vi "knownhosts_add.vi"() -> ()   [LabVIEW 2013]
doc: "Illustrates how to add a known host to the collection of known hosts."
uses:
  libssh2/libssh2_knownhost.ctl
  libssh2/Known Host Refnum.ctl
  libssh2/libssh2_init_default.vi
  libssh2/libssh2.lvlib
panel:
  out "error out":errorcluster
  out "known hosts":T1[](array[typedef])
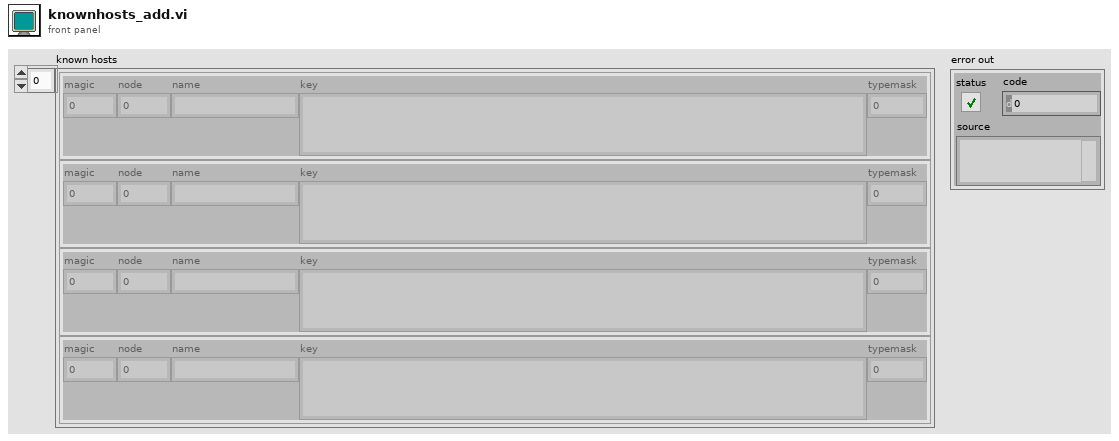
[diagram p1: front panel]
types:
  T1 = typedef "libssh2.lvlib/libssh2_knownhost.ctl" = cluster{"magic":u32, "node":u64, "name":string, "key":string, "typemask":i32}
  T2 = typedef "libssh2.lvlib/Known Host Refnum.ctl" = refnum<k1>
  T3 = typedef "libssh2.lvlib/Session Refnum.ctl" = refnum<k1>
  T4 = typedef "libssh2.lvlib/Known Host Collection Refnum.ctl" = refnum<k1>
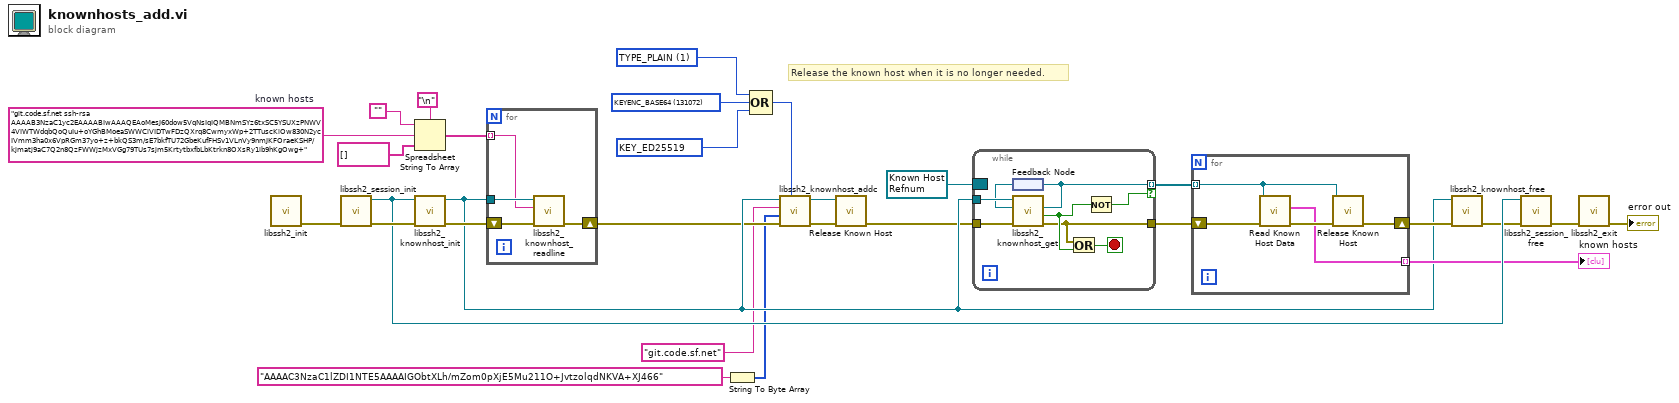
[diagram p0: block diagram]
diagram:
  w2 = 1835008 items=["TYPE_PLAIN"=1, "TYPE_SHA1"=2, "TYPE_CUSTOM"=3, "KEYENC_RAW"=65536, "KEYENC_BASE64"=131072, "KEY_RSA1"=262144, "KEY_SSHRSA"=524288, "KEY_SSHDSS"=786432, "KEY_ECDSA_256"=1048576, "KEY_ECDSA_384"=1310720, "KEY_ECDSA_521"=1572864, "KEY_ED25519"=1835008, "KEY_UNKNOWN"=3932160] ("typemask")
  w3 = 131072 items=["TYPE_PLAIN"=1, "TYPE_SHA1"=2, "TYPE_CUSTOM"=3, "KEYENC_RAW"=65536, "KEYENC_BASE64"=131072, "KEY_RSA1"=262144, "KEY_SSHRSA"=524288, "KEY_SSHDSS"=786432, "KEY_ECDSA_256"=1048576, "KEY_ECDSA_384"=1310720, "KEY_ECDSA_521"=1572864, "KEY_ED25519"=1835008, "KEY_UNKNOWN"=3932160] ("typemask")
  w4 = 1 items=["TYPE_PLAIN"=1, "TYPE_SHA1"=2, "TYPE_CUSTOM"=3, "KEYENC_RAW"=65536, "KEYENC_BASE64"=131072, "KEY_RSA1"=262144, "KEY_SSHRSA"=524288, "KEY_SSHDSS"=786432, "KEY_ECDSA_256"=1048576, "KEY_ECDSA_384"=1310720, "KEY_ECDSA_521"=1572864, "KEY_ED25519"=1835008, "KEY_UNKNOWN"=3932160] ("typemask")
  w19 = "git.code.sf.net ssh-rsa AAAAB3NzaC1yc2EAAAABIwAAAQEAoMesJ60dow5VqNsIqIQMBNmSYz6txSC5YSUXzPNWV4VIWTWdqbQoQuIu+oYGhBMoeaSWWCiVIDTwFDzQXrq8CwmyxWp+2TTuscKiOw830N2ycIVmm3ha0x6VpRGm37yo+z+bkQS3m/sE7bkfTU72GbeKufFHSv1VLnVy9nmJKFOraeKSHP/kjmatj9aC7Q2n8QzFWWjzMxVGg79TUs7sjm5KrtytbxfbLbKtrkn8OXsRy1ib9hKgOwg+"  # known hosts
  w21 = T2 refnum items=["Host"] ("next")
  # "Release the known host when it is no longer needed."
  n1 = call-poly "libssh2_init.vi"() -> ("error out"=w29:errorcluster)  [unwired: 11 in]
  n2 = call "libssh2_session_init.vi"("error in (no error)"=w29) -> ("error out"=w28:errorcluster, "session"=w27:T3)  [unwired: 9 in]
  n3 = Spreadsheet String To Array(delimiter (Tab)="\n", format string="", spreadsheet string=w19, array type (2D Dbl)=string[] []) -> (array=w18:string[])
  n4 = call "libssh2_knownhost_init.vi"("error in (no error)"=w28, "session"=w27) -> ("error out"=w24:errorcluster, "known hosts collection"=w11:T4)  [unwired: 8 in]
  n5 = for {
    tunnel: w11 -> [w31]
    tunnel: w18 -> [w30] mode=indexing
    shift-right: [w32] -> w10
    shift-left: w24 -> [w33]
    n6 = call "libssh2_knownhost_readline.vi"("error in (no error)"=w33, "line"=w30, "known hosts collection"=w31) -> ("error out"=w32:errorcluster)  [unwired: 8 in]
  }
  n7 = String To Byte Array(string="AAAAC3NzaC1lZDI1NTE5AAAAIGObtXLh/mZom0pXjE5Mu211O+JvtzolqdNKVA+XJ466" ("hostname")) -> (unsigned byte array=w7:u8[])
  n8 = Compound Arithmetic op=OR(w4, w3, w2) -> (w1:i32)
  n9 = call "libssh2_knownhost_addc.vi"("typemask"=w1, "error in (no error)"=w10, "key"=w7, "hostname"="git.code.sf.net", "known hosts collection"=w11) -> ("error out"=w12:errorcluster, "known host"=w5:T2)  [unwired: 5 in]
  n10 = call "Release Known Host.vi"("error in (no error)"=w12, "known host"=w5) -> ("error out"=w6:errorcluster)  [unwired: 9 in]
  n11 = while {
    tunnel: w6 -> [w41]
    tunnel: [w35] -> w23
    tunnel: w11 -> [w40]
    border: w21 -> [_]
    tunnel: [w37] -> w20 mode=indexing if=w34
    stop <- w39 stop-if-true
    n12 = feedback #1() -> (w38:T2)
    n13 = call "libssh2_knownhost_get.vi"("error in (no error)"=w41, "previous"=w38, "known hosts collection"=w40) -> ("error out"=w35:errorcluster, "end reached"=w36:bool, "next"=w37:T2)  [unwired: 6 in]
    n14 = feedback-in #1(w37) -> ()
    n15 = Or(x=w35, y=w36) -> (x .or. y?=w39:bool)
    n16 = Not(x=w36) -> (.not. x?=w34:bool)
  }
  n17 = for {
    shift-right: [w46] -> w22
    shift-left: w23 -> [w45]
    tunnel: w20 -> [w42] mode=indexing
    tunnel: [w43] -> w14 mode=indexing
    n18 = call "Read Known Host Data.vi"("error in (no error)"=w45, "known host"=w42) -> ("error out"=w44:errorcluster, "known host data"=w43:T1)  [unwired: 8 in]
    n19 = call "Release Known Host.vi"("error in (no error)"=w44, "known host"=w42) -> ("error out"=w46:errorcluster)  [unwired: 9 in]
  }
  "known hosts" <- w14
  n20 = call "libssh2_knownhost_free.vi"("error in (no error)"=w22, "known hosts collection"=w11) -> ("error out"=w26:errorcluster)  [unwired: 9 in]
  n21 = call "libssh2_session_free.vi"("error in (no error)"=w26, "session"=w27) -> ("error out"=w25:errorcluster)  [unwired: 9 in]
  n22 = call "libssh2_exit.vi"("error in (no error)"=w25) -> ("error out"=→"error out":errorcluster)  [unwired: 10 in]
